vi "Create DSFGroup.vi"(8 "error in (no error)":errorcluster, 9 "DSFGroup info":T1, 10 "id":string, 11 "DSFGroup in":refnum<class "DSFGroup.lvclass">) -> (0 "error out":errorcluster, 3 "DSFGroup out":refnum<class "DSFGroup.lvclass">)   [LabVIEW 2017, in "DSFGroup.lvclass"]
uses:
  DSFGroup.lvclass
  DSFTiming/DSFTiming.lvclass
  DSFGroup.lvclass/DSFGroup.ctl
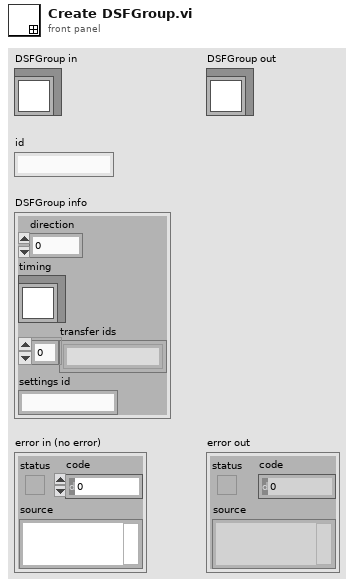
[diagram p1: front panel]
types:
  T1 = cluster{"direction":i32, "timing":refnum<class "DSFTiming.lvclass">, "transfer ids":string[], "settings id":string}
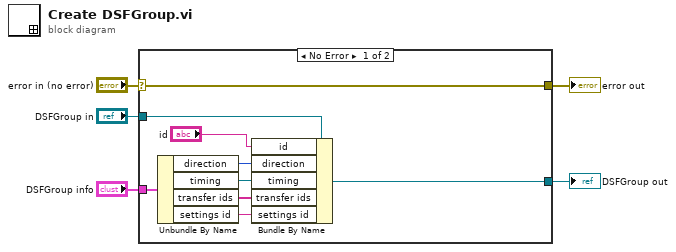
[diagram p0: block diagram]
diagram:
  n1 = case shown="No Error" "error in (no error)" {
    selector: "error in (no error)" -> [w13 w16]
    tunnel: [w13 w16] -> w4
    tunnel: [w12 w15] -> w2
    tunnel: "DSFGroup in" -> [w14 w15]
    tunnel: "DSFGroup info" -> [w10 _]
    frame No Error {
      n2 = Unbundle By Name(w10) -> ("direction"=w9:i32, "timing"=w8:refnum<class "DSFTiming.lvclass">, "transfer ids"=w7:string[], "settings id"=w6:string)
      n3 = Bundle By Name(cluster=w14, "id"="id", "direction"=w9, "timing"=w8, "transfer ids"=w7, "settings id"=w6) -> (w12:refnum<class "DSFGroup.lvclass">)
    }
    frame Error {
    }
  }
  "error out" <- w4
  "DSFGroup out" <- w2
